vi "RT Main.vi"() -> ()   [LabVIEW 2013]
uses:
  Cluser.ctl
  <vilib>/rvi/interface/common/niFpgaWaitOnOcc.vi
  <vilib>/FPGAPlugInAG/myRIO-1900/niLvFpga_Open_myRIO-1900.vi
  <vilib>/rvi/interface/common/dynamic/niFpgaDynamicAddResources.vi
  <vilib>/myRIO/Common/Instrument Driver Framework/Utilities/vis/FPGA Ref Manager.vi
  <vilib>/Utility/error.llb/Error Cluster From Error Code.vi
  <vilib>/rvi/errors/niLvFpgaAdjustHostInterfaceError.vi
  <vilib>/FPGAPlugInAG/Dynamic/niLvFpga_Close_Dynamic.vi
  <vilib>/rvi/interface/nirviOpenFPGA/nirviOpenFPGA.xnode
  FPGA Bitfiles/LEDMatrix4_FPGATarget_myRIO-1900Custom_r1aLzQW2H5E.lvbitx
  <vilib>/rvi/interface/nirviMethod/nirviMethod.xnode
  <vilib>/rvi/interface/nirviReadWriteControl/nirviReadWriteControl.xnode
  <vilib>/rvi/interface/nirviCloseFPGA/nirviCloseFPGA.xnode
  <vilib>/myRIO/Instrument Drivers/Utilities/Utilities.lvlib
  <vilib>/rvi/errors/niLvFpgaMergeErrorWithErrorCode.vi
  <vilib>/FPGAPlugInAG/Dynamic/niLvFpga_ConfigureFifo_Dynamic.vi
  <vilib>/FPGAPlugInAG/Dynamic/niLvFpga_StartFifo_Dynamic.vi
  NiFpgaLv.dll
  <vilib>/rvi/interface/Simulation/niFpgaSimulationCallBeginRW.vi
  <vilib>/FPGAPlugInAG/Dynamic/niLvFpga_StopFifo_Dynamic.vi
panel:
  in  "Tab Control":T1(tab)
  in  "Fill Colors":bool
  in  "Cluster":T2={"x start"=0, "x end"=15, "y start"=0, "y end"=15, "Fill Color"=16711871, "BG Color"=255}
  in  "Brightness":u8=50 min=1 step=1
  out "LED Matrix 2":picture
  in  "Display Oval":bool
  in  "Cluster":T2={"x start"=10, "x end"=30, "y start"=3, "y end"=12, "Fill Color"=393471, "BG Color"=10854655}
  in  "Brightness":u8=50 min=1 step=1
  out "LED Matrix":picture
  in  "Factor":dbl=2.5
  in  "Path (on myRio)":string="/home/admin/images/test.bmp"
  in  "Display Image":bool
  in  "Brightness":u8=50 max=100 step=1
  out "Rectangle":T3
  out "image depth":i32
  out "LED Matrix":picture
  in  "Factor":dbl=2.5 step=0.5
  in  "Display Text":bool
  in  "String":string="Hello"
  in  "Origin":cluster{"X":i32, "Y":i32}={"X"=2, "Y"=2}
  in  "Text BG Color":u32(colorbox)
  in  "Text Color":u32(colorbox)=16777215
  in  "Brightness":u8=50 min=1 step=1
  in  "Font, Size & Style":T4={"Desired Font (Application)"=enum."User-specified Font", "[User-specified Font]"={"Font Name"="", "Size"=10, "Strikeout?"=FALSE, "Italic?"=FALSE, "Underline?"=FALSE, "Outline?"=FALSE, "Shadow?"=FALSE, "Bold?"=FALSE, "Rotation Angle"=0.0}, "Horizontal Alignment"=0, "Vertical Alignment"=1} {"Vertical Alignment" items=["Bottom", "Top", "Baseline"]; "Horizontal Alignment" items=["Left", "Center", "Right"]; "[User-specified Font]"."Rotation Angle" format="%.2f"}
  in  "Rect BG Color":u32(colorbox)
  out "LED Matrix":picture
  in  "Factor":dbl=2.5
  in  "Brightness":u8=50 min=1 step=1
  in  "Pixel Test":bool
  in  "Period (ms)":u32=500
  in  "stop":bool
  in  "Color":u32(colorbox)=16777215
  out "error out":errorcluster
  out "SYS.RDY":bool
  out "Acceleration":T5(graph)
  in  "Stop Button":bool
  # "Overview: The myRIO Custom FPGA Project template acquires acceleration data from the onboard accelerometer and displays the changes of acceleration values in a waveform chart. The SYS.RDY indicator shows the FPGA status.\nRequirements: LabVIEW FPGA Module.\nInstructions:\n1. Check the myRIO target IP Address in the project and make sure the target IP Address is correct. \n2. Run the VI."
  # "Debugging Information"
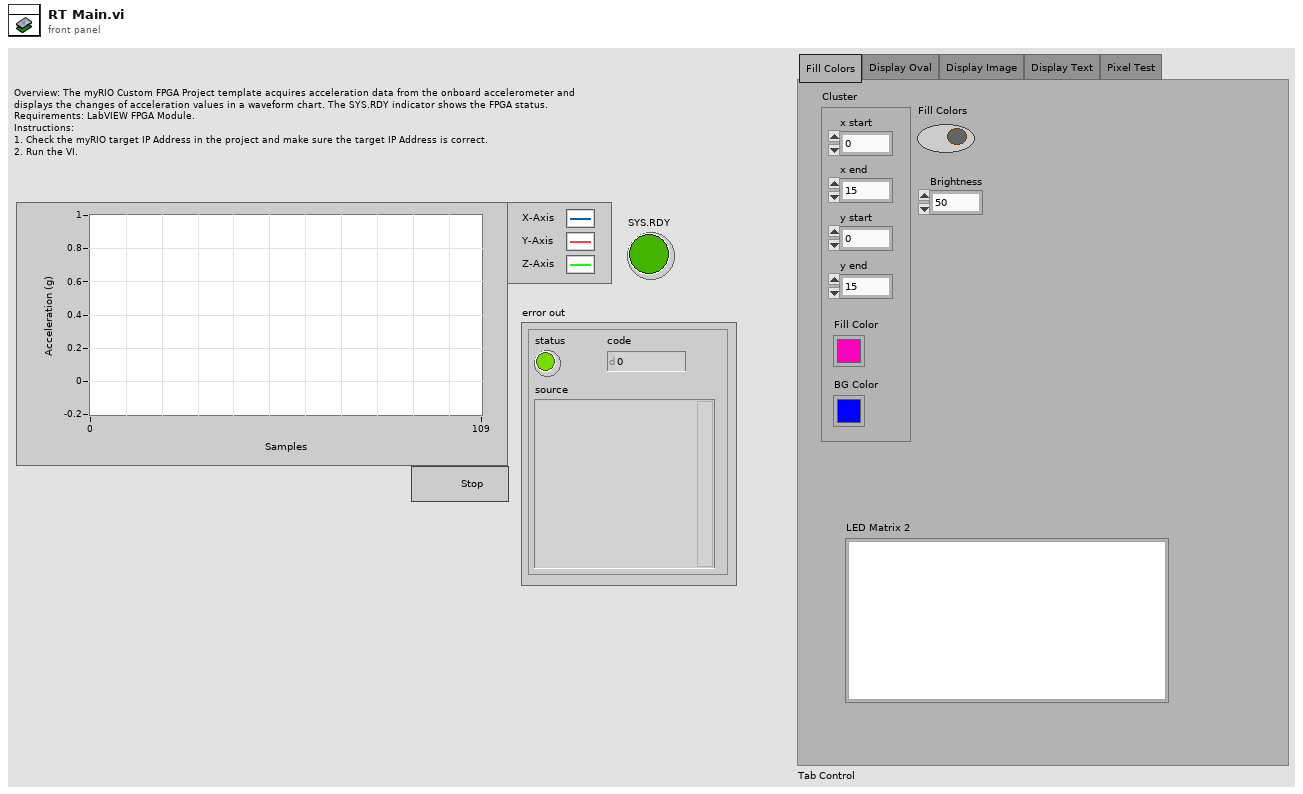
[diagram p1: front panel]
types:
  T1 = enum32{"Fill Colors", "Display Oval", "Display Image", "Display Text", "Pixel Test"}
  T2 = typedef "Cluser.ctl" = cluster{"x start":u16, "x end":u16, "y start":u16, "y end":u16, "Fill Color":u32, "BG Color":u32}
  T3 = cluster{"left":i16, "top":i16, "right":i16, "bottom":i16}
  T4 = cluster{"Desired Font (Application)":enum16{"User-specified Font", "Application Font", "System Font", "Dialog Font"}, "[User-specified Font]":cluster{"Font Name":string, "Size":i16, "Strikeout?":bool, "Italic?":bool, "Underline?":bool, "Outline?":bool, "Shadow?":bool, "Bold?":bool, "Rotation Angle":dbl}, "Horizontal Alignment":i16, "Vertical Alignment":i16}
  T5 = cluster{"X-Axis":dbl, "Y-Axis":dbl, "Z-Axis":dbl}
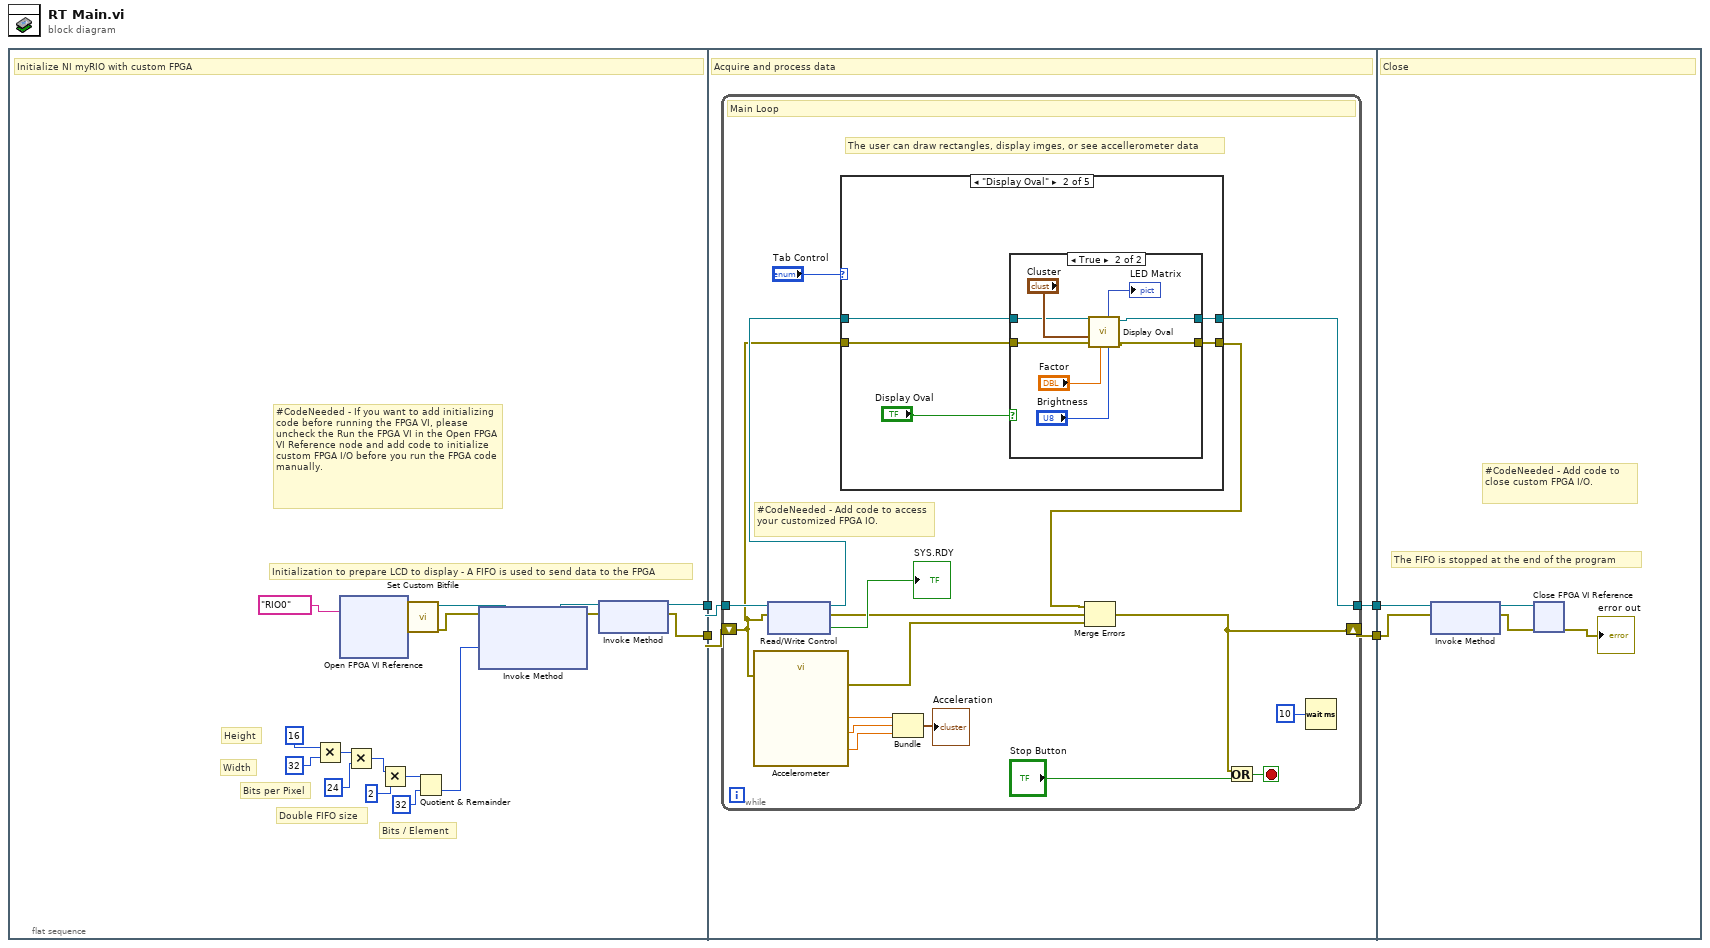
[diagram p0: block diagram]
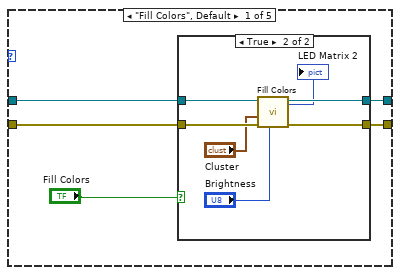
[diagram p2: hidden frame]
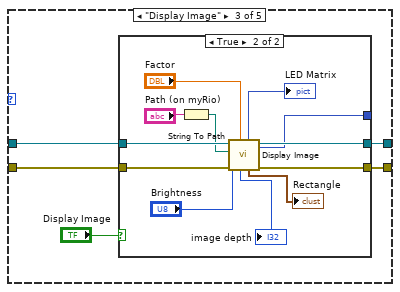
[diagram p5: hidden frame]
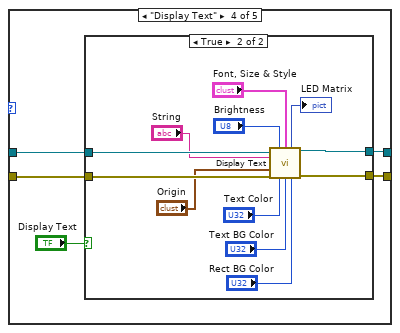
[diagram p7: hidden frame]
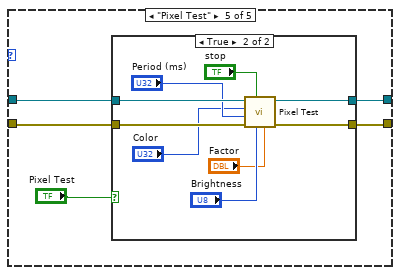
[diagram p9: hidden frame]
diagram:
  n1 = flat-sequence {
    tunnel: [w8] -> w4
    tunnel: [w9] -> w3
    tunnel: w4 -> [w26]
    tunnel: w3 -> [w25]
    tunnel: [w24] -> w2
    tunnel: [w23] -> w1
    tunnel: w2 -> [w129]
    tunnel: w1 -> [w127]
    frame #0 {
      # "Bits / Element"
      # "Double FIFO size"
      # "Bits per Pixel"
      # "Width"
      # "Height"
      # "Initialization to prepare LCD to display - A FIFO is used to send data to the FPGA"
      # "#CodeNeeded - If you want to add initializing code before running the FPGA VI, please uncheck the Run the FPGA VI in the Open FPGA VI Reference node and add code to initialize custom FPGA I/O before you run the FPGA code manually."
      # "Initialize NI myRIO with custom FPGA"
      n2 = Multiply(x=u32 16 ("Requested Depth"), y=u32 32 ("Requested Depth")) -> (x*y=w17:u32)
      n3 = xnode "Open FPGA VI Reference"("resource name"=tag "RIO0") -> ("FPGA VI Reference Out"=w6:refnum<k20>, "error out"=w22:errorcluster)  [unwired: 1 in]
      n4 = Multiply(x=w17, y=u32 24 ("Requested Depth")) -> (x*y=w15:u32)
      n5 = Multiply(x=w15, y=u32 2 ("Requested Depth")) -> (x*y=w13:u32)
      n6 = call <vilib>:"Set Custom Bitfile.vi"("error in (no error)"=w22, "Customized FPGA Reference in"=w6) -> ("error out"=w10:errorcluster, "Customized FPGA Reference out"=w11:refnum<k20>)  [unwired: 8 in]
      n7 = Quotient & Remainder(x=w13, y=u32 32 ("Requested Depth")) -> (floor(x/y)=w7:u32)  [unwired: 1 out]
      n8 = xnode "Invoke Method"("FPGA VI Reference In"=w11, "error in"=w10, "Requested Depth"=w7) -> ("FPGA VI Reference Out"=w21:refnum<k20>, "error out"=w20:errorcluster)  [unwired: 1 out]
      n9 = xnode "Invoke Method"("FPGA VI Reference In"=w21, "error in"=w20) -> ("FPGA VI Reference Out"=w9:refnum<k20>, "error out"=w8:errorcluster)
    }
    frame #1 {
      # "Acquire and process data"
      n10 = while {
        tunnel: w25 -> [w41]
        tunnel: [w29] -> w24
        shift-right: [w37] -> w23
        shift-left: w26 -> [w28]
        stop <- w42 stop-if-true
        # "The user can draw rectangles, display imges, or see accellerometer data"
        # "#CodeNeeded - Add code to access your customized FPGA IO."
        # "Main Loop"
        n11 = call "Accelerometer"("error in (no error)"=w28) -> ("X-Axis"=w36:dbl, "Y-Axis"=w34:dbl, "Z-Axis"=w35:dbl, "error out"=w32:errorcluster)  [unwired: 23 in]
        n12 = xnode "Read/Write Control"("FPGA VI Reference In"=w41, "error in"=w28) -> ("FPGA VI Reference Out"=w30:refnum<k20>, "error out"=w38:errorcluster, "SYS.RDY"=→"SYS.RDY":bool)
        n13 = case shown="\"Display Oval\"" "Tab Control" {
          tunnel: w30 -> [w48 w62 w75 w94 w113]
          tunnel: w28 -> [w47 w61 w74 w93 w112]
          tunnel: [w46 w60 w77 w92 w111] -> w29
          tunnel: [w45 w59 w76 w91 w110] -> w27
          frame "Fill Colors", Default {
            n14 = case shown="True" "Fill Colors" {
              tunnel: [w50 w57] -> w46
              tunnel: [w49 w56] -> w45
              tunnel: w48 -> [w50 w55]
              tunnel: w47 -> [w49 w54]
              frame False {
              }
              frame True {
                n15 = call "Fill Colors.vi"("Dim"="Brightness", "error in (no error)"=w54, "Cluster"="Cluster", "Refnum in"=w55) -> ("error out"=w56:errorcluster, "Refnum out"=w57:refnum<k20>, "LED Matrix"=→"LED Matrix 2":picture)  [unwired: 5 in]
              }
            }
          }
          frame "Display Oval" {
            n16 = case shown="True" "Display Oval" {
              tunnel: [w64 w68] -> w60
              tunnel: [w63 w69] -> w59
              tunnel: w62 -> [w64 w71]
              tunnel: w61 -> [w63 w70]
              frame False {
              }
              frame True {
                n17 = call "Display Oval.vi"("Brightness"="Brightness", "Factor"="Factor", "error in (no error)"=w70, "Cluster"="Cluster", "Refnum in"=w71) -> ("error out"=w69:errorcluster, "Refnum out"=w68:refnum<k20>, "LED Matrix"=→"LED Matrix":picture)  [unwired: 4 in]
              }
            }
          }
          frame "Display Image" {
            n18 = case shown="True" "Display Image" {
              tunnel: [w79 w90] -> w77
              tunnel: [w78 w89] -> w76
              tunnel: w75 -> [w79 w88]
              tunnel: w74 -> [w78 w87]
              tunnel: [_ w81] -> _
              frame False {
              }
              frame True {
                n19 = String To Path(string="Path (on myRio)") -> (path=w84:path)
                n20 = call "Display Image.vi"("Factor"="Factor", "error in (no error)"=w87, "Brightness"="Brightness", "path to BMP file on myRio local filesystem"=w84, "Refnum in"=w88) -> ("error out"=w89:errorcluster, "Refnum out"=w90:refnum<k20>, "Rectangle"=→"Rectangle":T3, "LED Matrix"=w81:picture, "image depth"=→"image depth":i32)  [unwired: 2 in]
                "LED Matrix" <- w81
              }
            }
          }
          frame "Display Text" {
            n21 = case shown="True" "Display Text" {
              tunnel: [w97 w108] -> w92
              tunnel: [w96 w106] -> w91
              tunnel: w94 -> [w97 w109]
              tunnel: w93 -> [w96 w107]
              frame False {
              }
              frame True {
                n22 = call "Display Text.vi"("Refnum in"=w109, "Brightness"="Brightness", "Font, Size & Style"="Font, Size & Style", "String"="String", "Origin"="Origin", "error in (no error)"=w107, "Text Color"="Text Color", "Text BG Color"="Text BG Color", "Rect BG Color"="Rect BG Color") -> ("LED Matrix"=→"LED Matrix":picture, "Refnum out"=w108:refnum<k20>, "error out"=w106:errorcluster)  [unwired: 4 in]
              }
            }
          }
          frame "Pixel Test" {
            n23 = case shown="True" "Pixel Test" {
              tunnel: [w116 w124] -> w111
              tunnel: [w115 w123] -> w110
              tunnel: w113 -> [w116 w125]
              tunnel: w112 -> [w115 w122]
              frame False {
              }
              frame True {
                n24 = call "Pixel Test.vi"("Factor"="Factor", "Brightness"="Brightness", "stop"="stop", "error in (no error)"=w122, "Period (ms)"="Period (ms)", "Color"="Color", "Refnum in"=w125) -> ("error out"=w123:errorcluster, "Refnum out"=w124:refnum<k20>)  [unwired: 3 in]
              }
            }
          }
        }
        n25 = Bundle("X-Axis"=w36, "Y-Axis"=w34, "Z-Axis"=w35) -> (→"Acceleration":T5)  [unwired: 1 in]
        n26 = Merge Errors(w27, w38, w32) -> (w37:errorcluster)
        n27 = Or(x=w37, y="Stop Button") -> (x .or. y?=w42:bool)
        n28 = Wait (ms)(milliseconds to wait=u32 10) -> ()  [unwired: 1 out]
      }
    }
    frame #2 {
      # "The FIFO is stopped at the end of the program"
      # "#CodeNeeded - Add code to close custom FPGA I/O."
      # "Close"
      n29 = xnode "Invoke Method"("FPGA VI Reference In"=w129, "error in"=w127) -> ("FPGA VI Reference Out"=w128:refnum<k20>, "error out"=w126:errorcluster)
      n30 = xnode "Close FPGA VI Reference"("FPGA VI Reference In"=w128, "error in"=w126) -> ("error out"=→"error out":errorcluster)
    }
  }
